vi "loop helper.vi"(8 "error in (no error)":errorcluster, 11 "Template in":refnum<class "Template.lvclass">) -> ()   [LabVIEW 2020, in "Template.lvlib" / "Template.lvclass"]
doc: "Executes the programmatic behaviors of the application defined by the user events cluster\nThe error found on any method is first ingested here through the New Error event\nUser can choose to execute interrupt messages by implementing code in the interrupt routine override and setting the timeout in ms in the configuration file\nThis should not be used as an User Interface or to handle any UI implementation"
uses:
  Template.lvclass
  C:/Program Files/National Instruments/LabVIEW 2020/vi.lib/ActorFramework/Actor/Actor.lvclass
  Template.lvclass/Template.ctl
  <vilib>/ActorFramework/Actor/Actor.lvclass/Actor.ctl
  <vilib>/ActorFramework/Message Enqueuer/Message Enqueuer.lvclass/Message Enqueuer.ctl
  <vilib>/ActorFramework/Message Enqueuer/Message Priority.ctl
  typedefs/actor configuration.ctl
  typedefs/shared actor configuration.ctl
  typedefs/resource config/device configuration cluster.ctl
  typedefs/resource config/single resource cluster.ctl
  Template Messages/update actor configuration Msg/update actor configuration Msg.lvclass/update actor configuration Msg.ctl
  Template Messages/fire error object Msg/fire error object Msg.lvclass/fire error object Msg.ctl
  Template Messages/process error Msg/process error Msg.lvclass/process error Msg.ctl
  interfaces/Error Interface Messages/process error Msg/process error Msg.lvclass/process error Msg.ctl
  <vilib>/ActorFramework/Message Enqueuer/Enqueue.vi
  tools/check if root actor.vi
  share error upstream.vi
  acessors/Read Nested Actors.vi
  Template Messages/process error Msg/Send process error.vi
  interfaces/Error Interface Messages/process error Msg/Send process error.vi
  <vilib>/ActorFramework/Message Enqueuer/Init from Existing Queue.vi
  <vilib>/ActorFramework/Message Enqueuer/Equals Not A Refnum.vi
  <vilib>/ActorFramework/Actor/Read Caller Enqueuer.vi
  Template Messages/fire error object Msg/Send fire error object.vi
  Template Messages/launch nested actors Msg/launch nested actors Msg.lvclass
  C:/Program Files/National Instruments/LabVIEW 2020/vi.lib/ActorFramework/Message/Message.lvclass
  Template Messages/interrupt routine Msg/interrupt routine Msg.lvclass
  Template Messages/update actor configuration Msg/update actor configuration Msg.lvclass
  Template Messages/fire error object Msg/fire error object Msg.lvclass
  Template Messages/process error Msg/process error Msg.lvclass
  interfaces/Error Interface Messages/process error Msg/process error Msg.lvclass
  <vilib>/ActorFramework/Message Priority Queue/Priority Enqueue.vi
  interfaces/Error Interface/Error/append time stamp.vi
  interfaces/Error Interface/Error/build error object.vi
  <vilib>/ActorFramework/Message Enqueuer/Message Enqueuer.lvclass
  <vilib>/ActorFramework/Actor/Actor.lvclass
panel:
  # "This should not be used as an User Interface or to handle any UI implementation"
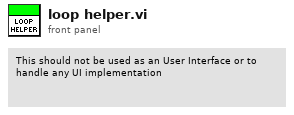
[diagram p1: front panel]
types:
  T1 = typedef "Actor Framework.lvlib/Message Enqueuer.lvclass/Message Priority.ctl" = enum16{"Low", "Normal", "High"}
  T2 = typedef "Template.lvlib/Template.lvclass/base actor events.ctl" = cluster{"Stop Actor":refnum<user-event>, "New Error":refnum<user-event>, "New Settings":refnum<user-event>}
  T3 = typedef "Template.lvlib/Template.lvclass/actor configuration.ctl" = cluster{"GlobalConfiguration":T4, "DeviceConfiguration":T5}
  T4 = typedef "Template.lvlib/Template.lvclass/shared actor configuration.ctl" = cluster{"DeviceFamily":string, "WriteData":bool, "BufferSize_samples":i32, "SyncDevice":bool, "ExecuteInterruptRoutine":bool, "InterruptRoutineTimeout_ms":i32}
  T5 = typedef "Template.lvlib/Template.lvclass/device configuration cluster.ctl" = cluster{"DeviceSpecificName":string, "HardwareReference":string, "UsedResources":T6[]}
  T6 = typedef "Template.lvlib/Template.lvclass/single resource cluster.ctl" = cluster{"ResourceLocation":string, "ResourceData":variant}
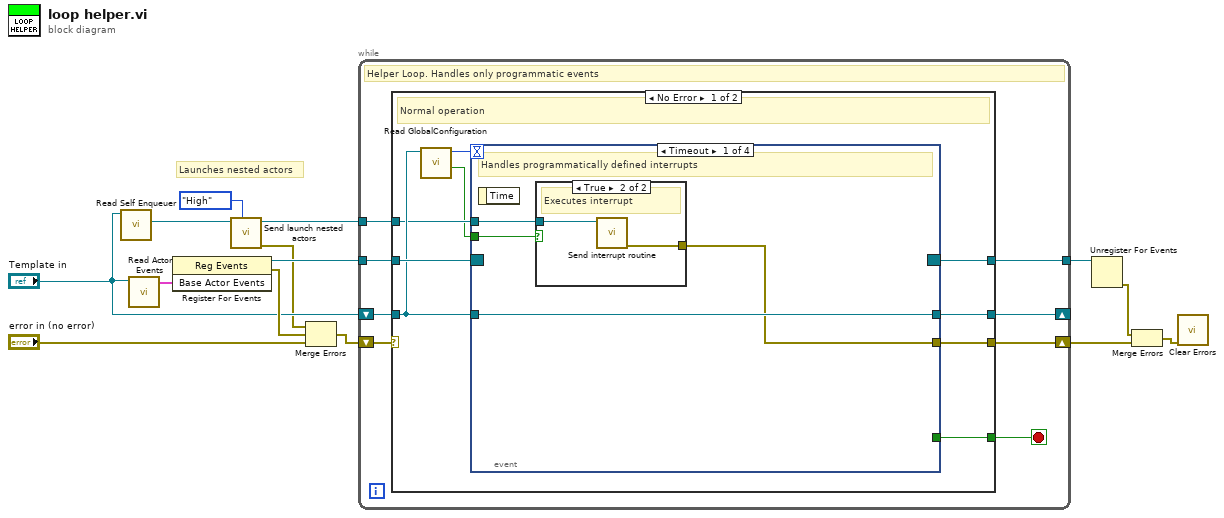
[diagram p0: block diagram]
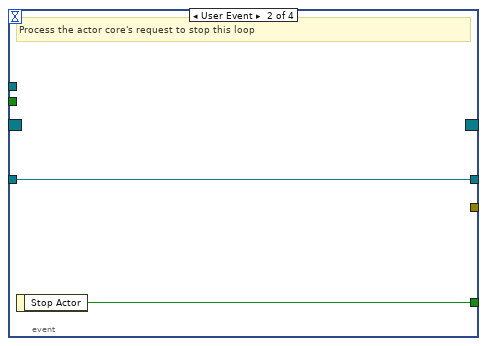
[diagram p3: hidden frame]
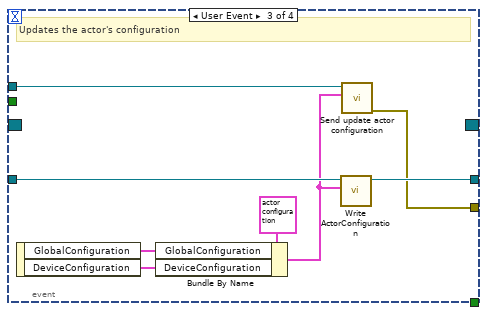
[diagram p4: hidden frame]
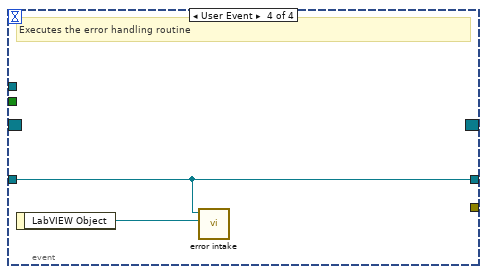
[diagram p5: hidden frame]
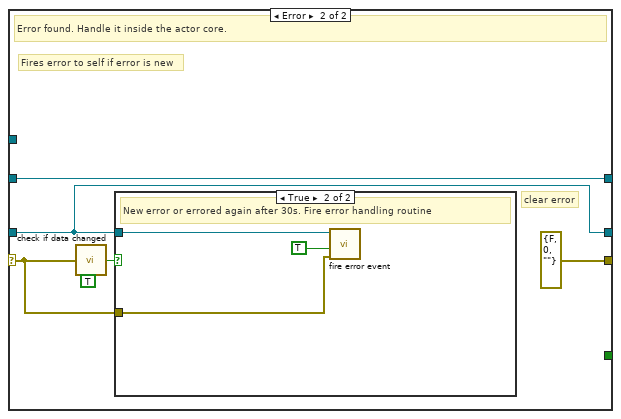
[diagram p6: hidden frame]
diagram:
  # "Launches nested actors"
  n1 = call <vilib>:"Read Self Enqueuer.vi"("Actor"="Template in") -> ("Self Enqueuer"=w4:refnum<class "Message Enqueuer.lvclass">)  [unwired: 10 in]
  n2 = call "Read Actor Events.vi"("Template in"="Template in") -> ("Base Actor Events"=w12:T2)  [unwired: 10 in]
  n3 = register-events(w12) -> (reference out=w13:refnum<event-registration>, error out=w6:errorcluster)  [unwired: 2 in]
  n4 = call "Send launch nested actors.vi"("Message Priority (Normal)"=Message_Priority."High", "Message Enqueuer"=w4) -> ("error out"=w1:errorcluster, "Message Enqueuer out"=w2:refnum<class "Message Enqueuer.lvclass">)  [unwired: 8 in]
  n5 = Merge Errors(w1, w6, "error in (no error)") -> (w7:errorcluster)
  n6 = while {
    tunnel: w13 -> [w22]
    shift-right: [w19] -> w11
    shift-left: w7 -> [w21]
    tunnel: [w20] -> w10
    shift-right: [w16] -> _
    shift-left: "Template in" -> [w17]
    tunnel: w2 -> [w15]
    stop <- w18 stop-if-true
    # "Helper Loop. Handles only programmatic events"
    n7 = case shown="No Error" w21 {
      selector: w21 -> [_ w51]
      tunnel: w22 -> [w31 w55]
      tunnel: [w30 w55] -> w20
      tunnel: [w24 errorcluster {"status"=FALSE, "code"=0, "source"=""} ("error IO")] -> w19
      tunnel: [w29 _] -> w18
      tunnel: w17 -> [w27 w52]
      tunnel: [w28 w52] -> w16
      tunnel: w15 -> [w25 _]
      frame No Error {
        # "Normal operation"
        n8 = call "Read GlobalConfiguration.vi"("Template in"=w27) -> ("ExecuteInterruptRoutine"=w23:bool, "InterruptRoutineTimeout"=w26:i32)  [unwired: 8 in, 1 out]
        n9 = event shown="[0] Timeout" {
          selector: w31 -> [_ _ _ _]
          dyn-events: [_ _ _ _] -> w30
          timeout: w26 -> [_ _ _ _]
          tunnel: [_ w39 _ _] -> w29
          tunnel: w27 -> [w35 w38 w45 w48]
          tunnel: [w35 w38 w44 w48] -> w28
          tunnel: w25 -> [w34 _ w42 _]
          tunnel: [w33 _ w40 _] -> w24
          tunnel: w23 -> [w32 _ _ _]
          event Timeout {
            # "Handles programmatically defined interrupts"
            n10 = event-data() -> ()  [unwired: 1 in, 1 out]
            n11 = case shown="True" w32 {
              tunnel: w34 -> [_ w37]
              tunnel: [_ w36] -> w33
              frame False {
                # "Do nothing on timeout"
              }
              frame True {
                # "Executes interrupt"
                n12 = call "Send interrupt routine.vi"("Message Enqueuer"=w37) -> ("error out"=w36:errorcluster)  [unwired: 9 in, 1 out]
              }
            }
          }
          event User Event {
            # "Process the actor core's request to stop this loop"
            n13 = event-data() -> ("Stop Actor"=w39:bool)  [unwired: 1 in]
          }
          event User Event {
            # "Updates the actor's configuration"
            n14 = event-data() -> ("GlobalConfiguration"=w47:T4, "DeviceConfiguration"=w46:T5)  [unwired: 1 in]
            n15 = Bundle By Name(cluster=T3 {"GlobalConfiguration"={"DeviceFamily"="", "WriteData"=FALSE, "BufferSize_samples"=-1, "SyncDevice"=FALSE, "ExecuteInterruptRoutine"=FALSE, "InterruptRoutineTimeout_ms"=-1}, "DeviceConfiguration"={"DeviceSpecificName"="MIPI_Camera", "HardwareReference"="PXIe-Slot2", "UsedResources"=[{"ResourceLocation"="FrontFacing", "ResourceData"=variant(string "Use this Variant to store your specific resource data.\nThis will be read from and written to with the JSON parsing API.\nIn the child implementation you can use the acessors provided to convert from the specific cluster to your own device's implementation")}]}} ("ActorConfiguration"), "GlobalConfiguration"=w47, "DeviceConfiguration"=w46) -> (w41:T3)
            n16 = call "Write ActorConfiguration.vi"("ActorConfiguration"=w41, "Template in"=w45) -> ("Template out"=w44:refnum<class "Template.lvclass">)  [unwired: 9 in]
            n17 = call "Send update actor configuration.vi"("ActorConfiguration"=w41, "Message Enqueuer"=w42) -> ("error out"=w40:errorcluster)  [unwired: 8 in, 1 out]
          }
          event User Event {
            # "Executes the error handling routine"
            n18 = event-data() -> ("LabVIEW Object"=w49:refnum<class>)  [unwired: 1 in]
            n19 = call "error intake.vi"("LabVIEW Object"=w49, "Template in"=w48) -> ()  [unwired: 10 in]
          }
        }
      }
      frame Error {
        # "clear error"
        # "Fires error to self if error is new"
        # "Error found. Handle it inside the actor core."
        n20 = call "check if data changed.vi"("Data"=w51, "Allow Report on Time? (F)"=TRUE) -> ("Data Changed?"=w54:bool)  [unwired: 3 in]
        n21 = case shown="True" w54 {
          tunnel: w52 -> [_ w58]
          tunnel: w51 -> [_ w56]
          frame False {
            # "Not a new error."
          }
          frame True {
            # "New error or errored again after 30s. Fire error handling routine"
            n22 = call "fire error event.vi"("Error to Process"=w56, "Report Error (F)"=TRUE, "Error Source"=w58) -> ()  [unwired: 9 in]
          }
        }
      }
    }
  }
  n23 = Unregister For Events(event registration refnum=w10) -> (error out=w8:errorcluster)  [unwired: 1 in]
  n24 = Merge Errors(w8, w11) -> (w9:errorcluster)
  n25 = call <vilib>:"Clear Errors.vi"("error in (no error)"=w9) -> ()  [unwired: 5 in, 2 out]
